vi "Main.vi"() -> ()   [LabVIEW 2020]
doc: "This template is for the Queued Message Handler design pattern.\n\nThe Event Handling Loop generates messages based on user interface actions.\n\nThe Message Handling Loop processes messages generated by the Event Handling Loop, or by other messages. The messages are string values, so new messages can be added easily to the Message Cases case structure in the Message Handling Loop. Each message cluster can also provide an optional value for Message Data, which is a variant that can be converted to whatever message-specific data is required."
uses:
  controls/UI Data.ctl
  controls/Arduino config -- cluster.ctl
  Arduino_stepper/Libraries/Arduino stepper/Support/Motor direction -- enum.ctl
  controls/Camera config parameters -- cluster.ctl
  <vilib>/userdefined/High Color/IMAQdx.ctl
  controls/FGV actions -- enum.ctl
  Arduino_stepper/Libraries/Arduino stepper/Support/COM params--typedef.ctl
  Arduino_stepper/Libraries/Arduino stepper/Support/Motor parameters.ctl
  support/Message Queue/Enqueue Message (Array).vi
  <vilib>/Utility/error.llb/Error Cluster From Error Code.vi
  <vilib>/ErrorRing/Error Ring.xnode
  support/Message Queue/Message Queue.lvlib
  support/User Event - Stop/User Event - Stop.lvlib
  Arduino_stepper/Libraries/Arduino stepper/Arduino stepper.lvlib
  Camera/Libraries/Camera/Camera.lvlib
panel:
  in  "Go to zero":bool
  in  "Mostrar video":bool
  in  "Set zero":bool
  in  "Step 2":dbl=1.0 caption="Paso" format="%#_g°"
  in  "CW Button":bool
  in  "CCW Button":bool
  out "Home?":bool
  in  "To Matlab":bool
  in  "Home":bool
  in  "Step":dbl=5.0 caption="Paso/captura" format="%#_g°"
  out "Image":T1(plugin-control)
  out "Cam connected?":bool
  out "Ard connected?":bool
  out "End-stops":cluster{"ES1":bool, "ES2":bool} caption="Finales de carrera"
  out "Posición actual":dbl format="%#_g°"
  in  "Ángulo":dbl=45.0 caption="Ángulo total" format="%#_g°"
  in  "Stop":bool
  in  "Start acquisition":bool
  in  "Settings":bool
  out "Status":string
  in  "Exit":bool
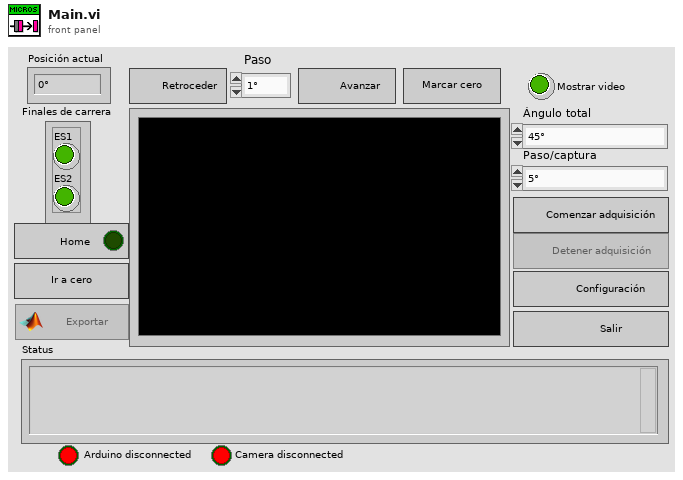
[diagram p1: front panel]
types:
  T1 = typedef "IMAQ Image.ctl" = refnum<image>
  T2 = typedef "UI Data.ctl" = cluster{"Status":string, "Arduino Mod ID":i32, "Arduino config":T3, "Current position":dbl, "End-stops":cluster{"ES1":bool, "ES2":bool}, "Direction":T4, "Camera Mod ID":i32, "Camera config":T5, "System ready?":bool, "Homing?":bool, "Path":path, "Path set?":bool, "Positions":dbl[], "Manual?":bool, "Zero":dbl, "Starting pos":dbl}
  T3 = typedef "Arduino config -- cluster.ctl" = cluster{"VISA resource":refnum<visa-resource-name>}
  T4 = typedef "Arduino stepper.lvlib/Motor direction -- enum.ctl" = enum8{"", "CW", "CCW"}
  T5 = typedef "Camera config parameters -- cluster.ctl" = cluster{"Camera session":T6, "VideoMode":u32}
  T6 = typedef "IMAQdx.ctl" = refnum<k21>
  T7 = typedef "Arduino stepper.lvlib/Broadcast Events--cluster.ctl" = cluster{"Module Did Init":refnum<user-event>, "Status Updated":refnum<user-event>, "Error Reported":refnum<user-event>, "Module Did Stop":refnum<user-event>, "Update Module Execution Status":refnum<user-event>, "Device connected":refnum<user-event>, "Data available":refnum<user-event>, "Info ready":refnum<user-event>, "Connection failed":refnum<user-event>, "Device disconected":refnum<user-event>, "End-position reached":refnum<user-event>, "End-stop reached":refnum<user-event>, "Home reached":refnum<user-event>}
  T8 = typedef "Camera.lvlib/Broadcast Events--cluster.ctl" = cluster{"Module Did Init":refnum<user-event>, "Status Updated":refnum<user-event>, "Error Reported":refnum<user-event>, "Module Did Stop":refnum<user-event>, "Update Module Execution Status":refnum<user-event>, "Helper Loop Status Updated":refnum<user-event>, "Camera connected":refnum<user-event>, "Camera Disconnected":refnum<user-event>, "Image acquired":refnum<user-event>, "Camera acquisition started":refnum<user-event>, "Camera acquisition stopped":refnum<user-event>}
  T9 = typedef "Message Queue.lvlib/All Message Queues.ctl" = cluster{"UI":refnum<queue>}
  T10 = typedef "FGV actions -- enum.ctl" = enum16{"Reset", "Get", "Increment"}
  T11 = enum8{"Enabled", "Disabled", "Disabled and Grayed Out"}
  T12 = typedef "Arduino stepper.lvlib/Motor parameters.ctl" = cluster{"Motor type":enum8{"", "Unipolar", "Bipolar"}, "Direction":T4, "Steps":u16, "Frequency (Hz)":u8, "Step type":enum8{"", "Half", "Full"}}
  T13 = cluster{"Position":i32, "End-stops":cluster{"ES1":bool, "ES2":bool}}
  T14 = typedef "Arduino stepper.lvlib/COM params--typedef.ctl" = cluster{"baud rate":u32, "data bits":u16, "parity":enum16{"None", "Odd", "Even", "Mark", "Space"}, "stop bits":u16, "flow control":u16}
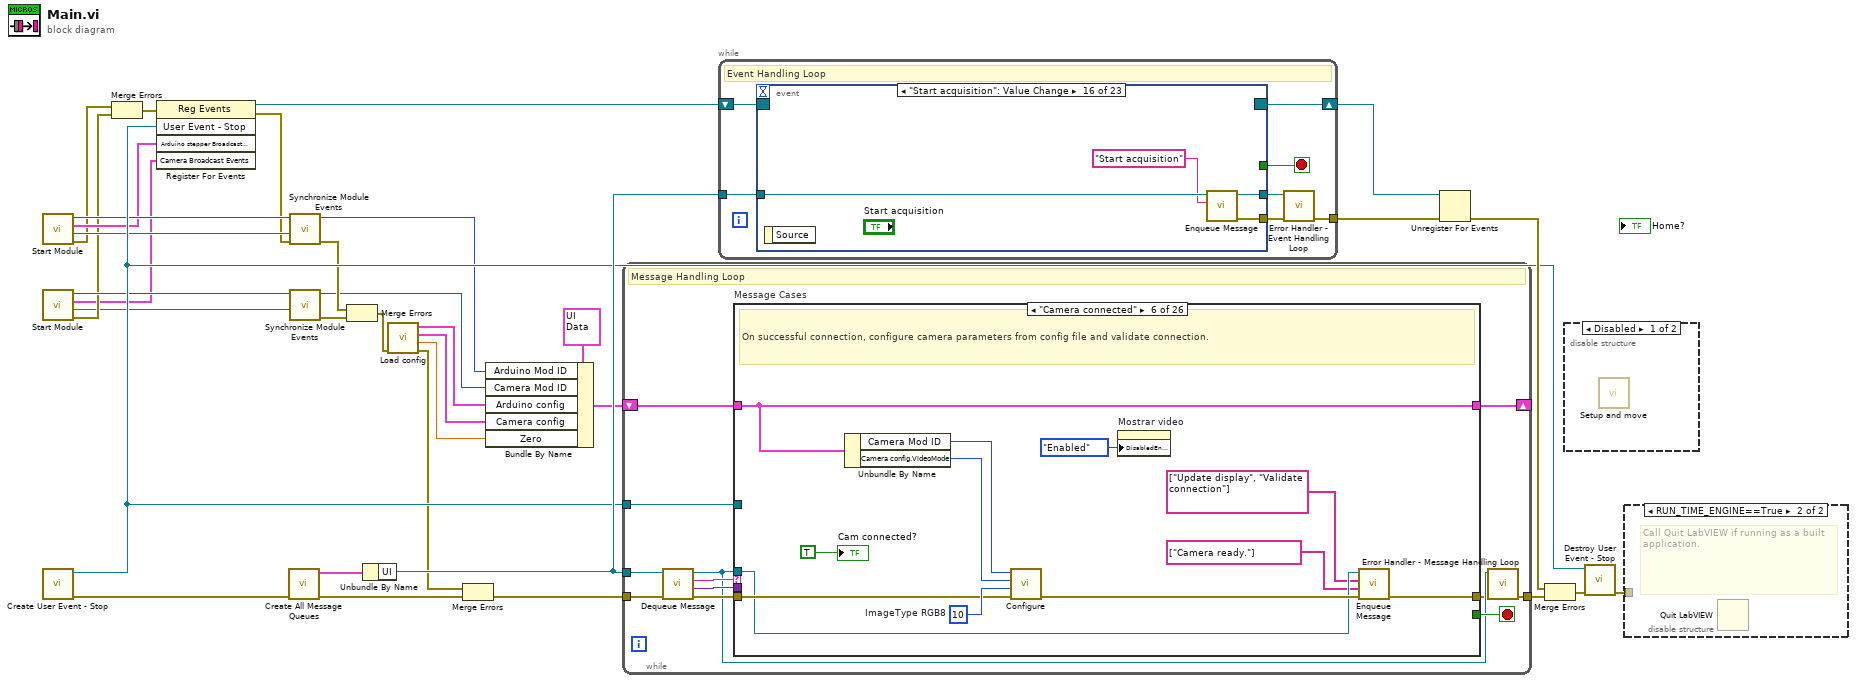
[diagram p0: block diagram]
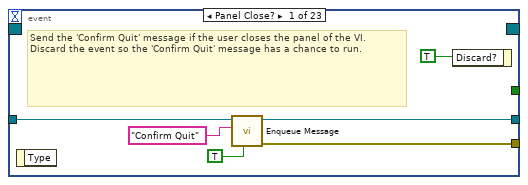
[diagram p4: hidden frame]
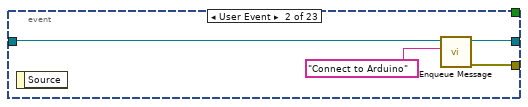
[diagram p5: hidden frame]
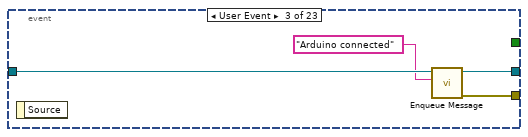
[diagram p6: hidden frame]
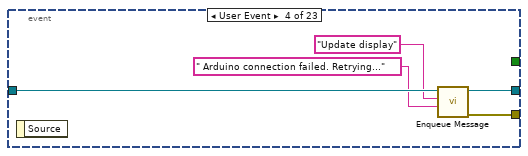
[diagram p7: hidden frame]
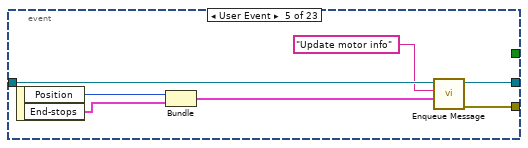
[diagram p8: hidden frame]
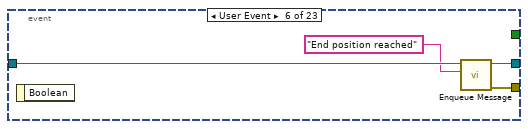
[diagram p9: hidden frame]
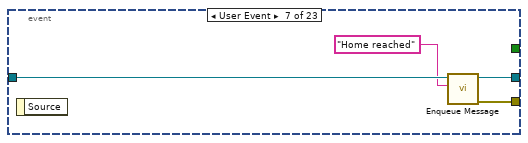
[diagram p10: hidden frame]
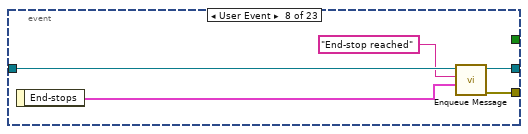
[diagram p11: hidden frame]
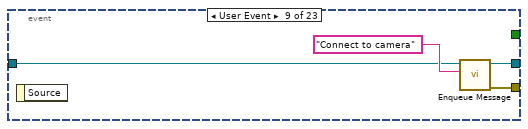
[diagram p12: hidden frame]
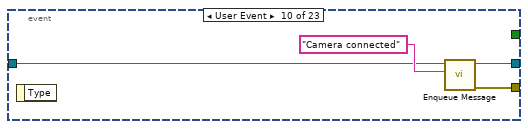
[diagram p13: hidden frame]
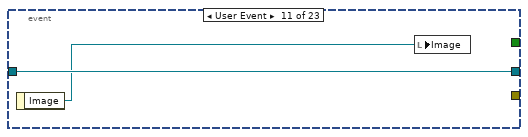
[diagram p14: hidden frame]
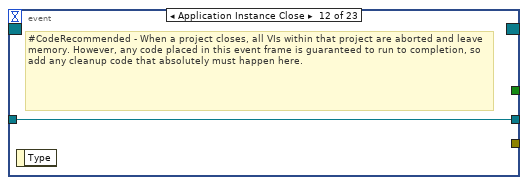
[diagram p15: hidden frame]
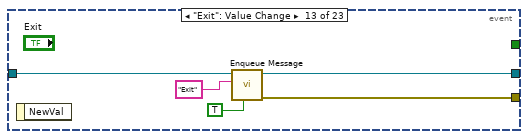
[diagram p16: hidden frame]
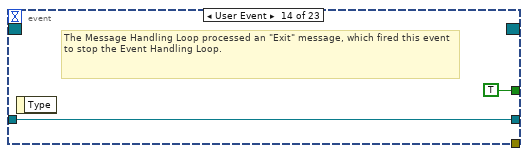
[diagram p17: hidden frame]
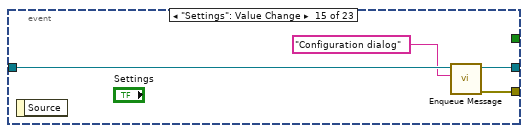
[diagram p18: hidden frame]
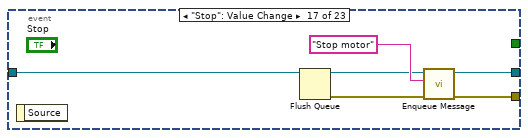
[diagram p19: hidden frame]
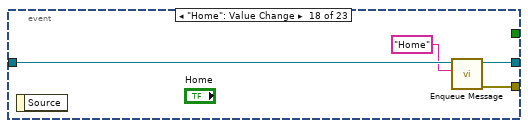
[diagram p20: hidden frame]
diagram:
  n1 = call "Start Module.vi"() -> ("error out"=w9:errorcluster, "Wait for Event Sync?"=w20:bool, "Arduino stepper Broadcast Events"=w21:T7, "Module ID"=w22:i32)  [unwired: 8 in]
  n2 = call "Start Module.vi"() -> ("error out"=w6:errorcluster, "Wait for Event Sync?"=w4:bool, "Camera Broadcast Events"=w5:T8, "Module ID"=w7:i32)  [unwired: 8 in]
  n3 = call "Create User Event - Stop.vi"() -> ("error out"=w31:errorcluster, "User Event - Stop"=w24:refnum<user-event>)  [unwired: 10 in]
  n4 = Merge Errors(w9, w6) -> (w10:errorcluster)
  n5 = register-events(error in=w10, w24, w21, w5) -> (reference out=w25:refnum<event-registration>, error out=w15:errorcluster)  [unwired: 1 in]
  n6 = call "Create All Message Queues.vi"("error in (no error)"=w31) -> ("error out"=w11:errorcluster, "Message Queues out"=w34:T9)  [unwired: 9 in]
  n7 = call "Synchronize Module Events.vi"("error in"=w15, "Wait for Event Sync?"=w20, "Module ID in"=w22) -> ("error out"=w14:errorcluster, "Module ID out"=w17:i32)  [unwired: 7 in]
  n8 = call "Synchronize Module Events.vi"("Wait for Event Sync?"=w4, "Module ID in"=w7) -> ("error out"=w8:errorcluster, "Module ID out"=w3:i32)  [unwired: 8 in]
  n9 = Merge Errors(w14, w8) -> (w13:errorcluster)
  n10 = Unbundle By Name(w34) -> ("UI"=w32:refnum<queue>)
  n11 = call "Load config.vi"("error in (no error)"=w13) -> ("error out"=w12:errorcluster, "Zero"=w1:dbl, "Camera config"=w2:T5, "Arduino config"=w16:T3)  [unwired: 7 in]
  n12 = Merge Errors(w12, w11) -> (w23:errorcluster)
  n13 = Bundle By Name(cluster=T2 {"Status"="", "Arduino Mod ID"=0, "Arduino config"={"VISA resource"=""}, "Current position"=0.0, "End-stops"={"ES1"=FALSE, "ES2"=FALSE}, "Direction"=enum."CW", "Camera Mod ID"=0, "Camera config"={"Camera session"="", "VideoMode"=0}, "System ready?"=FALSE, "Homing?"=FALSE, "Path"=path "", "Path set?"=FALSE, "Positions"=[], "Manual?"=FALSE, "Zero"=0.0, "Starting pos"=0.0} ("Data Cluster"), "Arduino Mod ID"=w17, "Camera Mod ID"=w3, "Arduino config"=w16, "Camera config"=w2, "Zero"=w1) -> (w18:T2)
  n14 = while {
    tunnel: w32 -> [w38]
    shift-right: [w45] -> _
    shift-left: w18 -> [w46]
    tunnel: w24 -> [w43]
    tunnel: w23 -> [w42]
    tunnel: [w36] -> w33
    stop <- w44 stop-if-true
    # "Message Handling Loop"
    n15 = call "Dequeue Message.vi"("error in (no error)"=w42, "Message Queue"=w38) -> ("error out"=w41:errorcluster, "Message Data"=w39:variant, "Message"=w40:string, "dup Message Queue"=w37:refnum<queue>)  [unwired: 6 in]
    n16 = case "Message Cases" shown="\"Camera connected\"" w40 {
      selector: w40 -> [_ _ _ _ _ _ _ _ _ _ _ _ _ _ _ _ _ _ _ _ _ _ _ _ _ w646]
      tunnel: w37 -> [w59 _ w76 w98 w121 w128 w141 w170 w199 w215 _ w283 w321 w371 w387 w415 w464 w497 _ w547 _ _ _ w624 w645 _]
      tunnel: w41 -> [w52 w75 w84 w104 w116 w134 w143 w176 w204 _ w271 w294 w319 w374 w394 w409 w470 w490 w528 w549 w599 w607 w621 w628 w640 _]
      tunnel: [w61 w63 w79 w100 w122 w129 w142 w173 w200 w218 w270 w285 w324 w372 w388 w420 w463 w498 w527 w548 w598 w606 w615 w626 w643 w647] -> w35
      tunnel: w46 -> [w57 w67 w77 w105 w119 w133 w140 w172 w196 w209 w268 w281 w323 w379 w386 w418 w469 w503 w518 w544 w597 w605 w620 w627 w634 w648]
      tunnel: [w56 w65 w77 w105 w118 w133 w137 w171 w195 w217 w269 w280 w322 w379 w385 w417 w468 w502 w517 w543 w597 w605 w620 w627 w634 w648] -> w45
      tunnel: [_ _ _ _ _ _ _ _ _ _ _ _ _ _ _ _ _ _ _ _ _ _ _ _ TRUE _] -> w44
      tunnel: w39 -> [_ w74 _ _ _ _ _ _ _ _ w266 w293 _ _ w392 _ w466 _ _ _ _ w602 w619 _ w637 _]
      tunnel: w43 -> [_ _ _ _ _ _ _ _ _ _ _ _ _ _ _ _ _ _ _ _ _ _ _ _ w642 _]
      frame "Initialize" {
        w49 = FALSE ("System ready?")
        w47 = T11."Disabled and Grayed Out" ("Disabled")
        # "Initialize - All initialization work should take place in this message, since other loops can potentially enqueue messages that execute immediately after this one."
        n17 = call "Image name -- FGV.vi"("error in (no error)"=w52, "Action"=FGV_actions_--_enum."Reset", "Base name"=path "Image_") -> ("error out"=w51:errorcluster)  [unwired: 7 in, 1 out]
        n18 = property on="Start acquisition" class="Bool"("DisabledEnum"=w47) -> ()  [unwired: 2 in, 2 out]
        n19 = property on="To Matlab" class="Bool"("DisabledEnum"=w47) -> ()  [unwired: 2 in, 2 out]
        n20 = property on="Go to zero" class="Bool"("DisabledEnum"=w47) -> ()  [unwired: 2 in, 2 out]
        n21 = property on="Stop" class="Bool"("DisabledEnum"=w47) -> ()  [unwired: 2 in, 2 out]
        n22 = property on="Show/stop video" class="Bool (strict)"("DisabledEnum"=w47, "Value"=FALSE ("Mostrar video")) -> ()  [unwired: 2 in, 2 out]
        n23 = call-poly "Enqueue Message.vi"("error in (no error)"=w51, "Message Data"="Initializing..." ("Initial Message"), "Message"="Update Display", "Message Queue"=w59) -> ("error out"=w61:errorcluster)  [unwired: 6 in, 1 out]
        n24 = Bundle By Name(cluster=w57, "Positions"=dbl[] [0.0], "Current position"=0.0, "Homing?"=w49, "System ready?"=w49, "Path set?"=w49, "Manual?"=w49) -> (w56:T2)
        n25 = local write "Ard connected?"(w49) -> ()
        n26 = local write "Cam connected?"(w49) -> ()
        n27 = local write "Home?"(w49) -> ()
      }
      frame "Update Display" {
        # "Update Display - Convert the message data to a string to display in the Data Display indicator."
        n28 = Variant To Data(error in=w75, type="", Variant=w74) -> (data=w68:string, error out=w64:errorcluster)
        n29 = Unbundle By Name(w67) -> ("Status"=w70:string)
        n30 = Format Date/Time String(time format string (%c)="%d/%m/%y %H:%M:%S%3u") -> (date/time string=w69:string)  [unwired: 2 in]
        n31 = Format Into String(format string="%s: %s\\n", initial string=w70, w69, w68) -> (resulting string=w66:string)  [unwired: 1 in, 1 out]
        "Status" <- w66
        n32 = property on="Status" class="Str"(error in=w64, "Text.Scroll Position"=u32 10000) -> (error out=w63:errorcluster)  [unwired: 1 in, 1 out]
        n33 = Bundle By Name(cluster=w67, "Status"=w66) -> (w65:T2)
      }
      frame "Connect to Arduino" {
        w85 = T14 {"baud rate"=115200, "data bits"=8, "parity"=enum."None", "stop bits"=10, "flow control"=0}  # COM params
        # "Try two reconnections to Arduino. If connection is not successful, call configuration dialog."
        n34 = Unbundle By Name(w77) -> ("Arduino Mod ID"=w78:i32, "Arduino config.VISA resource"=w83:refnum<visa-resource-name>)
        n35 = for {
          N: 2 -> [_]
          tunnel: w85 -> [w96]
          tunnel: w78 -> [w94]
          tunnel: w83 -> [w93]
          shift-right: [w92] -> w80
          shift-left: w84 -> [w95]
          tunnel: [w91] -> w81
          stop <- w91 stop-if-true
          n36 = call "Connect.vi"("error in"=w95, "COM params"=w96, "VISA resource"=w93, "Module ID"=w94) -> ("error out"=w92:errorcluster, "Connected?"=w91:bool)  [unwired: 5 in, 1 out]
        }
        n37 = case shown="False" w81 {
          tunnel: w80 -> [w86 w90]
          tunnel: [w86 w89] -> w79
          tunnel: w78 -> [_ _]
          tunnel: w76 -> [_ w87]
          frame True {
            # "Connection successful."
          }
          frame False {
            # "Could not connect."
            n38 = call-poly "Enqueue Message.vi"("error in (no error)"=w90, "Message"="Configuration dialog", "Message Queue"=w87) -> ("error out"=w89:errorcluster)  [unwired: 7 in, 1 out]
          }
        }
      }
      frame "Connect to camera" {
        w103 = FALSE  # Simulate?
        n39 = Unbundle By Name(w105) -> ("Camera Mod ID"=w101:i32, "Camera config.Camera session"=w97:T6)
        n40 = call "Connect USB.vi"("error in"=w104, "Simulate?"=w103, "Camera session"=w97, "Module ID"=w101) -> ("error out"=w102:errorcluster, "Connected?"=w99:bool)  [unwired: 5 in, 1 out]
        n41 = case shown="False" w99 {
          tunnel: w102 -> [w108 w110]
          tunnel: [w107 w110] -> w100
          tunnel: w98 -> [w106 _]
          frame False {
            # "Connection to camera not made."
            n42 = call-poly "Enqueue Message.vi"("error in (no error)"=w108, "Message"="Configuration dialog", "Message Queue"=w106) -> ("error out"=w107:errorcluster)  [unwired: 7 in, 1 out]
          }
          frame True {
            # "Connection successful."
          }
        }
      }
      frame "Arduino connected" {
        # "On successful connection, update end-stops status and go to validate connection."
        n43 = Unbundle By Name(w119) -> ("Arduino Mod ID"=w120:i32)
        n44 = call "Wait ms.vi"("error in (no error)"=w116, "milliseconds to wait"=u32 100) -> ("error out"=w115:errorcluster)  [unwired: 9 in]
        n45 = call "Read end-stops.vi"("error in"=w115, "Module ID"=w120) -> ("error out"=w123:errorcluster, "End-stops"=w117:cluster{"ES1":bool, "ES2":bool})  [unwired: 7 in, 1 out]
        n46 = local write "End-stops"(w117) -> ()
        n47 = Bundle By Name(cluster=w119, "End-stops"=w117) -> (w118:T2)
        n48 = call-poly "Enqueue Message.vi"("error in (no error)"=w123, "Message Data Array"=string[] ["Arduino ready."] ("Message"), "Message Array"=string[] ["Update display", "Validate connection"] ("Message"), "Message Queue"=w121) -> ("error out"=w122:errorcluster)  [unwired: 6 in, 1 out]
        "Ard connected?" <- TRUE ("Ard connected?")
      }
      frame "Camera connected" {
        w135 = u32 10  # ImageType RGB8
        # "On successful connection, configure camera parameters from config file and validate connection."
        n49 = Unbundle By Name(w133) -> ("Camera Mod ID"=w131:i32, "Camera config.VideoMode"=w132:u32)
        n50 = call "Configure.vi"("error in"=w134, "ImageType"=w135, "VideoMode"=w132, "Module ID"=w131) -> ("error out"=w130:errorcluster)  [unwired: 7 in]
        n51 = property on="Mostrar video" class="Bool (strict)"("DisabledEnum"=T11."Enabled" ("Disabled")) -> ()  [unwired: 2 in, 2 out]
        n52 = call-poly "Enqueue Message.vi"("error in (no error)"=w130, "Message Data Array"=string[] ["Camera ready."] ("Message"), "Message Array"=string[] ["Update display", "Validate connection"] ("Message"), "Message Queue"=w128) -> ("error out"=w129:errorcluster)  [unwired: 6 in, 1 out]
        "Cam connected?" <- TRUE ("Cam connected?")
      }
      frame "Validate connection" {
        # "If both devices connection is successful and system not marked as ready,  set ready flag and home motor position. Otherwise, keep waiting for validation."
        n53 = local read "Cam connected?"() -> (w145:bool)
        n54 = local read "Ard connected?"() -> (w146:bool)
        n55 = Unbundle By Name(w140) -> ("Arduino Mod ID"=w136:i32, "System ready?"=w139:bool)
        n56 = Not(x=w139) -> (.not. x?=w138:bool)
        n57 = Compound Arithmetic op=AND(w138, w146, w145) -> (w144:bool)
        n58 = case shown="True" w144 {
          tunnel: w143 -> [w148 w153]
          tunnel: [w148 w162] -> w142
          tunnel: w141 -> [_ w160]
          tunnel: w140 -> [w147 w157]
          tunnel: [w147 w156] -> w137
          tunnel: w136 -> [_ w149]
          frame False {
          }
          frame True {
            w154 = T11."Disabled and Grayed Out" ("Disabled")
            n59 = call "Read end-stops.vi"("error in"=w153, "Module ID"=w149) -> ("error out"=w152:errorcluster, "End-stops"=w150:cluster{"ES1":bool, "ES2":bool})  [unwired: 7 in, 1 out]
            n60 = property on="Start acquisition" class="Bool"("DisabledEnum"=T11."Enabled" ("Disabled")) -> ()  [unwired: 2 in, 2 out]
            n61 = property on="Home" class="Bool"("DisabledEnum"=w154) -> ()  [unwired: 2 in, 2 out]
            n62 = property on="Stop" class="Bool"(error in=w152, "DisabledEnum"=w154) -> (error out=w151:errorcluster)  [unwired: 1 in, 1 out]
            n63 = Bundle By Name(cluster=w157, "System ready?"=TRUE, "End-stops"=w150) -> (w156:T2)
            n64 = call-poly "Enqueue Message.vi"("error in (no error)"=w151, "Message Data Array"=string[] ["System ready."] ("Message"), "Message Array"=string[] ["Update display", "Home"] ("Message"), "Message Queue"=w160) -> ("error out"=w162:errorcluster)  [unwired: 6 in, 1 out]
          }
        }
      }
      frame "Configuration dialog" {
        n65 = Unbundle By Name(w172) -> ("Camera Mod ID"=w165:i32, "Arduino Mod ID"=w169:i32, "Arduino config"=w175:T3, "Camera config"=w164:T5, "Zero"=w163:dbl)
        n66 = call "Config dialog.vi"("error in (no error)"=w176, "Camera config in"=w164, "Arduino config in"=w175) -> ("error out"=w174:errorcluster, "Cancelled?"=w168:bool, "Camera config out"=w166:T5, "Arduino config out"=w167:T3)  [unwired: 5 in]
        n67 = case shown="False" w168 {
          tunnel: w174 -> [w188 w193]
          tunnel: [w186 w192] -> w173
          tunnel: w170 -> [w185 w191]
          tunnel: w169 -> [w187 _]
          tunnel: w167 -> [w183 _]
          tunnel: w166 -> [w182 _]
          tunnel: w165 -> [w179 _]
          tunnel: w163 -> [w177 _]
          frame False {
            # "Disconnect devices and apply new configuration"
            n68 = call "Disconnect.vi"("error in"=w188, "Module ID"=w187) -> ("error out"=w181:errorcluster)  [unwired: 9 in]
            n69 = call "Disconnect.vi"("error in"=w181, "Module ID"=w179) -> ("error out"=w180:errorcluster)  [unwired: 9 in]
            n70 = call "Save config.vi"("error in (no error)"=w180, "Zero"=w177, "Camera config"=w182, "Arduino config"=w183) -> ("error out"=w184:errorcluster)  [unwired: 7 in]
            n71 = call-poly "Enqueue Message.vi"("error in (no error)"=w184, "Message Array"=string[] ["Connect to Arduino", "Connect to camera"] ("Message"), "Message Queue"=w185) -> ("error out"=w186:errorcluster)  [unwired: 7 in, 1 out]
          }
          frame True {
            # "Config dialog cancelled. Do nothing."
            n72 = call-poly "Enqueue Message.vi"("error in (no error)"=w193, "Message Data"="Configuration cancelled." ("Message"), "Message"="Update display", "Message Queue"=w191) -> ("error out"=w192:errorcluster)  [unwired: 6 in, 1 out]
          }
        }
        n73 = Bundle By Name(cluster=w172, "Arduino config"=w167, "Camera config"=w166) -> (w171:T2)
      }
      frame "Save zero" {
        n74 = Unbundle By Name(w196) -> ("Arduino config"=w203:T3, "Camera config"=w202:T5)
        n75 = local read "Posición actual"() -> (w194:dbl)
        n76 = call "Save config.vi"("error in (no error)"=w204, "Zero"=w194, "Camera config"=w202, "Arduino config"=w203) -> ("error out"=w201:errorcluster)  [unwired: 7 in]
        n77 = Bundle By Name(cluster=w196, "Zero"=w194) -> (w195:T2)
        n78 = call-poly "Enqueue Message.vi"("error in (no error)"=w201, "Message Data"="Starting position updated." ("Message"), "Message"="Update display", "Message Queue"=w199) -> ("error out"=w200:errorcluster)  [unwired: 6 in, 1 out]
      }
      frame "Start acquisition" {
        # "Call file dialog to set a path for all images. If path is not set, do not acquire.\nMove motor only if move conditions are correct. Save first image at 0° of movement."
        n79 = Unbundle By Name(w209) -> ("Arduino Mod ID"=w214:i32, "Camera Mod ID"=w207:i32, "Path"=w212:path, "Path set?"=w210:bool, "End-stops"=w205:cluster{"ES1":bool, "ES2":bool})
        n80 = local read "Home?"() -> (w206:bool)
        n81 = call "Set path.vi"("Path set?"=w210, "Path in"=w212) -> ("error out"=w213:errorcluster, "cancelled?"=w211:bool, "Path out"=w208:path)  [unwired: 7 in]
        n82 = case shown="False" w211 {
          tunnel: [w235 w256] -> w218
          tunnel: [w234 w252] -> w217
          tunnel: Motor_direction_--_enum."CCW" ("Direction") -> [w232 _]
          tunnel: w215 -> [w231 w255]
          tunnel: w214 -> [w228 _]
          tunnel: w213 -> [w227 w257]
          tunnel: w209 -> [w226 w252]
          tunnel: w208 -> [w223 _]
          tunnel: w207 -> [w222 _]
          tunnel: w206 -> [w221 _]
          tunnel: w205 -> [w219 _]
          frame False {
            # "Path is set correctly. Start aquisition."
            n83 = Bundle By Name(cluster=w226, "Path"=w223, "Path set?"=TRUE, "Manual?"=FALSE) -> (w224:T2)
            n84 = call "Check move conditions.vi"("Is Home?"=w221, "error in (no error)"=w227, "End-stops"=w219, "Direction"=w232) -> ("error out"=w233:errorcluster, "String"=w229:string, "Move?"=w230:bool)  [unwired: 5 in]
            n85 = case shown="True" w230 {
              tunnel: [w241 w251] -> w235
              tunnel: w228 -> [_ _]
              tunnel: [w236 w245] -> w234
              tunnel: w233 -> [w240 w250]
              tunnel: w232 -> [_ w247]
              tunnel: w231 -> [w239 w249]
              tunnel: w229 -> [w237 _]
              tunnel: w224 -> [w236 w246]
              tunnel: w222 -> [_ _]
              frame False {
                # "Move conditions not met"
                n86 = call-poly "Enqueue Message.vi"("error in (no error)"=w240, "Message Data"=w237, "Message"="Update Display", "Message Queue"=w239) -> ("error out"=w241:errorcluster)  [unwired: 6 in, 1 out]
              }
              frame True {
                # "Start moving"
                n87 = local read "Posición actual"() -> (w242:dbl)
                n88 = Build Array(w242) -> (w243:dbl[])
                n89 = Bundle By Name(cluster=w246, "End-stops"=cluster{"ES1":bool, "ES2":bool} {"ES1"=FALSE, "ES2"=FALSE}, "Positions"=w243, "Starting pos"=w242) -> (w245:T2)
                n90 = call-poly "Enqueue Message.vi"("error in (no error)"=w250, "Message Data"=w247, "Message"="Begin movement", "Message Queue"=w249) -> ("error out"=w251:errorcluster)  [unwired: 6 in, 1 out]
              }
            }
          }
          frame True {
            # "Path not set. Do nothing."
            n91 = call-poly "Enqueue Message.vi"("error in (no error)"=w257, "Message Data"="Path not selected or empty. Stopping acquisition." ("Message"), "Message"="Update Display", "Message Queue"=w255) -> ("error out"=w256:errorcluster)  [unwired: 6 in, 1 out]
          }
        }
      }
      frame "Begin movement" {
        w274 = T11."Enabled" ("Disabled")
        w259 = T11."Disabled and Grayed Out" ("Disabled")
        n92 = Variant To Data(error in=w271, type=Motor_direction_--_enum."CCW" ("Direction"), Variant=w266) -> (data=w264:T4, error out=w261:errorcluster)
        n93 = Unbundle By Name(w268) -> ("Arduino Mod ID"=w267:i32, "Path"=w262:path, "Camera Mod ID"=w260:i32)
        n94 = call "Get and save image.vi"("error in (no error)"=w261, "Camera Mod ID"=w260, "Path"=w262) -> ("error out"=w276:errorcluster, "Image out"=→"Image":T1)  [unwired: 7 in]
        n95 = call "Setup and move.vi"("Motor params"=T12 {"Motor type"=enum."Unipolar", "Direction"=enum."CW", "Steps"=1000, "Frequency (Hz)"=127, "Step type"=enum."Full"}, "error in (no error)"=w276, "Ángulo"="Step", "Direction"=w264, "Arduino Mod ID"=w267) -> ("error out"=w270:errorcluster)  [unwired: 6 in]
        n96 = Bundle By Name(cluster=w268, "Homing?"=FALSE, "Direction"=w264) -> (w269:T2)
        n97 = local write "Home?"(FALSE ("Home?")) -> ()
        n98 = property on="Home" class="Bool"("DisabledEnum"=w274) -> ()  [unwired: 2 in, 2 out]
        n99 = property on="Stop" class="Bool"("DisabledEnum"=w274) -> ()  [unwired: 2 in, 2 out]
        n100 = property on="Start acquisition" class="Bool"("DisabledEnum"=w259) -> ()  [unwired: 2 in, 2 out]
        n101 = property on="Mostrar video" class="Bool (strict)"("DisabledEnum"=w259, "Value"=FALSE ("Mostrar video")) -> ()  [unwired: 2 in, 2 out]
      }
      frame "Jog" {
        n102 = Unbundle By Name(w281) -> ("Arduino Mod ID"=w287:i32, "End-stops"=w278:cluster{"ES1":bool, "ES2":bool})
        n103 = Variant To Data(error in=w294, type=Motor_direction_--_enum."CW" ("Direction"), Variant=w293) -> (data=w286:T4, error out=w292:errorcluster)
        n104 = disable-structure shown="Enabled" {
          disable-tunnel: w292 -> [w298 _]
          disable-tunnel: [w297 _] -> w291
          disable-tunnel: w287 -> [w296 _]
          disable-tunnel: [w295 w299] -> w279
          disable-tunnel: w278 -> [_ w299]
          frame Disabled {
            n105 = call "Read end-stops.vi"("error in"=w298, "Module ID"=w296) -> ("error out"=w297:errorcluster, "End-stops"=w295:cluster{"ES1":bool, "ES2":bool})  [unwired: 7 in, 1 out]
          }
          frame Enabled {
          }
        }
        n106 = local read "Home?"() -> (w282:bool)
        n107 = call "Check move conditions.vi"("Is Home?"=w282, "error in (no error)"=w291, "End-stops"=w279, "Direction"=w286) -> ("error out"=w288:errorcluster, "String"=w284:string, "Move?"=w289:bool)  [unwired: 5 in]
        n108 = case shown="True" w289 {
          tunnel: w288 -> [w304 w316]
          tunnel: w287 -> [_ w315]
          tunnel: w286 -> [_ w311]
          tunnel: [w305 w313] -> w285
          tunnel: w284 -> [w303 _]
          tunnel: w283 -> [w301 _]
          tunnel: w281 -> [w300 w308]
          tunnel: [w300 w312] -> w280
          frame False {
            n109 = call-poly "Enqueue Message.vi"("error in (no error)"=w304, "Message Data"=w303, "Message"="Update Display", "Message Queue"=w301) -> ("error out"=w305:errorcluster)  [unwired: 6 in, 1 out]
          }
          frame True {
            w306 = T11."Enabled" ("Disabled")
            n110 = call "Setup and move.vi"("Motor params"=T12 {"Motor type"=enum."Unipolar", "Direction"=enum."CW", "Steps"=1000, "Frequency (Hz)"=127, "Step type"=enum."Full"}, "error in (no error)"=w316, "Ángulo"="Step 2", "Direction"=w311, "Arduino Mod ID"=w315) -> ("error out"=w313:errorcluster)  [unwired: 6 in]
            n111 = property on="Home" class="Bool"("DisabledEnum"=w306) -> ()  [unwired: 2 in, 2 out]
            n112 = property on="Go to zero" class="Bool"("DisabledEnum"=w306) -> ()  [unwired: 2 in, 2 out]
            n113 = Bundle By Name(cluster=w308, "Manual?"=TRUE, "Direction"=w311, "End-stops"=cluster{"ES1":bool, "ES2":bool} {"ES1"=FALSE, "ES2"=FALSE}) -> (w312:T2)
            n114 = local write "Home?"(FALSE ("Home?")) -> ()
          }
        }
      }
      frame "Home" {
        # "If move conditions are met, move in CW direction 90 degrees or until ES1 is reached."
        n115 = Unbundle By Name(w323) -> ("Arduino Mod ID"=w320:i32)
        n116 = local read "Home?"() -> (w318:bool)
        n117 = disable-structure shown="Enabled" {
          disable-tunnel: [w337 w358] -> w324
          disable-tunnel: w323 -> [w336 w362]
          disable-tunnel: [w335 w360] -> w322
          disable-tunnel: w321 -> [w333 w357]
          disable-tunnel: w320 -> [w328 w363]
          disable-tunnel: w319 -> [w326 w368]
          disable-tunnel: w318 -> [w325 _]
          frame Disabled {
            w327 = Motor_direction_--_enum."CW" ("Direction")
            n118 = call "Read end-stops.vi"("error in"=w326, "Module ID"=w328) -> ("error out"=w330:errorcluster, "End-stops"=w329:cluster{"ES1":bool, "ES2":bool})  [unwired: 7 in, 1 out]
            n119 = call "Check move conditions.vi"("Is Home?"=w325, "error in (no error)"=w330, "End-stops"=w329, "Direction"=w327) -> ("error out"=w334:errorcluster, "String"=w331:string, "Move?"=w332:bool)  [unwired: 5 in]
            n120 = case shown="True" w332 {
              tunnel: [w342 w354] -> w337
              tunnel: w328 -> [_ w353]
              tunnel: w336 -> [w343 w352]
              tunnel: [w343 w351] -> w335
              tunnel: w334 -> [w341 w350]
              tunnel: w327 -> [_ w349]
              tunnel: w333 -> [w340 _]
              tunnel: w331 -> [w338 _]
              frame False {
                # "Move conditions not met"
                n121 = call-poly "Enqueue Message.vi"("error in (no error)"=w341, "Message Data"=w338, "Message"="Update Display", "Message Queue"=w340) -> ("error out"=w342:errorcluster)  [unwired: 6 in, 1 out]
              }
              frame True {
                w344 = 90.0  # Max angle
                # "Start moving"
                n122 = call "Setup and move.vi"("Motor params"=T12 {"Motor type"=enum."Unipolar", "Direction"=enum."CW", "Steps"=1000, "Frequency (Hz)"=255, "Step type"=enum."Full"}, "error in (no error)"=w350, "Ángulo"=w344, "Direction"=w349, "Arduino Mod ID"=w353) -> ("error out"=w354:errorcluster)  [unwired: 6 in]
                n123 = Bundle By Name(cluster=w352, "Direction"=w349, "Homing?"=TRUE) -> (w351:T2)
                n124 = property on="Start acquisition" class="Bool"("DisabledEnum"=T11."Disabled and Grayed Out" ("Disabled")) -> ()  [unwired: 2 in, 2 out]
                n125 = property on="Stop" class="Bool"("DisabledEnum"=T11."Enabled" ("Disabled")) -> ()  [unwired: 2 in, 2 out]
              }
            }
          }
          frame Enabled {
            w365 = 50  # Timeout
            n126 = call "Home.vi"("error in"=w368, "Module ID"=w363) -> ("error out"=w364:errorcluster)  [unwired: 9 in]
            n127 = Bundle By Name(cluster=w362, "Homing?"=TRUE) -> (w360:T2)
            n128 = call "Read port continuously.vi"("error in"=w364, "Timeout"=w365, "Module ID"=w363) -> ("error out"=w359:errorcluster)  [unwired: 8 in]
            n129 = call-poly "Enqueue Message.vi"("error in (no error)"=w359, "Message Data"="Homing..." ("Message"), "Message"="Update Display", "Message Queue"=w357) -> ("error out"=w358:errorcluster)  [unwired: 6 in, 1 out]
            n130 = property on="Start acquisition" class="Bool"("DisabledEnum"=T11."Disabled and Grayed Out" ("Disabled")) -> ()  [unwired: 2 in, 2 out]
            n131 = property on="Stop" class="Bool"("DisabledEnum"=T11."Enabled" ("Disabled")) -> ()  [unwired: 2 in, 2 out]
          }
        }
      }
      frame "Stop motor" {
        n132 = Unbundle By Name(w379) -> ("Arduino Mod ID"=w375:i32)
        n133 = call "Stop continuous reading.vi"("error in"=w374, "Module ID"=w375) -> ("error out"=w376:errorcluster)  [unwired: 9 in]
        n134 = call "Stop motor.vi"("error in"=w376, "Module ID"=w375) -> ("error out"=w373:errorcluster)  [unwired: 9 in]
        n135 = property on="Stop" class="Bool"("DisabledEnum"=T11."Disabled and Grayed Out" ("Disabled")) -> ()  [unwired: 2 in, 2 out]
        n136 = property on="Start acquisition" class="Bool"("DisabledEnum"=T11."Enabled" ("Disabled")) -> ()  [unwired: 2 in, 2 out]
        n137 = call-poly "Enqueue Message.vi"("error in (no error)"=w373, "Message Data"="Stop sent by user." ("Message"), "Message"="Update Display", "Message Queue"=w371) -> ("error out"=w372:errorcluster)  [unwired: 6 in, 1 out]
      }
      frame "Update motor info" {
        # "Get End-stop and position info from continous reading. If and end-stop is reached, stop movement."
        n138 = Variant To Data(error in=w394, type=T13 {"Position"=0, "End-stops"={"ES1"=FALSE, "ES2"=FALSE}} ("output cluster"), Variant=w392) -> (data=w391:T13, error out=w383:errorcluster)
        n139 = Unbundle By Name(w386) -> ("Current position"=w389:dbl, "Direction"=w380:T4)
        n140 = Unbundle By Name(w391) -> ("Position"=w390:i32, "End-stops"=w381:cluster{"ES1":bool, "ES2":bool})
        "End-stops" <- w381
        n141 = call "Calculate new position.vi"("error in (no error)"=w383, "Position from motor"=w390, "Direction"=w380, "Current position in"=w389) -> ("error out"=w382:errorcluster, "Position out"=w384:dbl)  [unwired: 6 in]
        "Posición actual" <- w384
        n142 = disable-structure shown="Enabled" {
          disable-tunnel: [w402 w408] -> w388
          disable-tunnel: w387 -> [w401 _]
          disable-tunnel: w382 -> [w400 w408]
          disable-tunnel: w381 -> [w399 _]
          disable-tunnel: w380 -> [w398 _]
          frame Disabled {
            n143 = local read "Home?"() -> (w395:bool)
            n144 = call "Check move conditions.vi"("Is Home?"=w395, "error in (no error)"=w400, "End-stops"=w399, "Direction"=w398) -> ("error out"=w397:errorcluster, "Move?"=w396:bool)  [unwired: 5 in, 1 out]
            n145 = case shown="True" w396 {
              tunnel: w397 -> [w403 w407]
              tunnel: [w405 w407] -> w402
              tunnel: w401 -> [w404 _]
              frame False {
                # "End-stop reached."
                n146 = call-poly "Enqueue Message.vi"("error in (no error)"=w403, "Message"="Stop motor", "Message Queue"=w404) -> ("error out"=w405:errorcluster)  [unwired: 7 in, 1 out]
              }
              frame True {
                # "Keep moving"
              }
            }
          }
          frame Enabled {
          }
        }
        n147 = Bundle By Name(cluster=w386, "Current position"=w384, "End-stops"=w381) -> (w385:T2)
      }
      frame "End position reached" {
        # "If end-position is reached, stop motor. If the motor is homing, change disable state of controls, otherwise check move condition."
        n148 = Unbundle By Name(w418) -> ("Manual?"=w414:bool, "Camera Mod ID"=w413:i32, "Arduino Mod ID"=w412:i32, "Homing?"=w419:bool, "Path"=w416:path)
        n149 = call "Stop continuous reading.vi"("error in"=w409, "Module ID"=w412) -> ("error out"=w410:errorcluster)  [unwired: 9 in]
        n150 = call "Stop motor.vi"("error in"=w410, "Module ID"=w412) -> ("error out"=w411:errorcluster)  [unwired: 9 in]
        n151 = case shown="False" w414 {
          tunnel: [w427 w450] -> w420
          tunnel: w419 -> [w426 _]
          tunnel: w418 -> [w425 w455]
          tunnel: [w424 w454] -> w417
          tunnel: w416 -> [_ _]
          tunnel: w415 -> [w423 _]
          tunnel: w411 -> [w422 w450]
          tunnel: w412 -> [w421 _]
          tunnel: w413 -> [_ _]
          frame False {
            # "Automatic movement. Check move conditions."
            n152 = case shown="False" w426 {
              tunnel: w422 -> [w429 w441]
              tunnel: [w436 w449] -> w427
              tunnel: w425 -> [w432 w446]
              tunnel: [w431 w444] -> w424
              tunnel: w423 -> [w435 w442]
              tunnel: w421 -> [_ _]
              frame False {
                # "Partial end-position. Check if system needs to keep moving."
                n153 = Unbundle By Name(w432) -> ("Positions"=w434:dbl[], "Current position"=w433:dbl)
                n154 = local read "Posición actual"() -> (w428:dbl)
                n155 = Build Array (concatenate)(w434, w433) -> (w430:dbl[])
                n156 = Bundle By Name(cluster=w432, "Positions"=w430, "Current position"=w428) -> (w431:T2)
                n157 = call-poly "Enqueue Message.vi"("error in (no error)"=w429, "Message Data Array"=string[] ["End-position reached."] ("Message"), "Message Array"=string[] ["Update Display", "Check move condition"] ("Message"), "Message Queue"=w435) -> ("error out"=w436:errorcluster)  [unwired: 6 in, 1 out]
              }
              frame True {
                w440 = T11."Enabled" ("Disabled")
                w443 = T11."Disabled and Grayed Out" ("Disabled")
                # "Zero position reached."
                n158 = property on="Start acquisition" class="Bool"("DisabledEnum"=w440) -> ()  [unwired: 2 in, 2 out]
                n159 = property on="Mostrar video" class="Bool (strict)"("DisabledEnum"=w440) -> ()  [unwired: 2 in, 2 out]
                n160 = property on="Home" class="Bool"("DisabledEnum"=w443) -> ()  [unwired: 2 in, 2 out]
                n161 = property on="Stop" class="Bool"("DisabledEnum"=w443) -> ()  [unwired: 2 in, 2 out]
                n162 = local read "Posición actual"() -> (w439:dbl)
                n163 = Bundle By Name(cluster=w446, "Homing?"=FALSE, "Current position"=w439) -> (w444:T2)
                n164 = call-poly "Enqueue Message.vi"("error in (no error)"=w441, "Message Data"="Zero position reached." ("Message"), "Message"="Update Display", "Message Queue"=w442) -> ("error out"=w449:errorcluster)  [unwired: 6 in, 1 out]
              }
            }
          }
          frame True {
            w451 = T11."Enabled" ("Disabled")
            # "Manual movement. Do nothing."
            n165 = Unbundle By Name(w455) -> ("Current position"=w453:dbl)
            n166 = Build Array(w453) -> (w452:dbl[])
            n167 = property on="Mostrar video" class="Bool (strict)"("DisabledEnum"=w451) -> ()  [unwired: 2 in, 2 out]
            n168 = property on="Start acquisition" class="Bool"("DisabledEnum"=w451) -> ()  [unwired: 2 in, 2 out]
            n169 = Bundle By Name(cluster=w455, "Positions"=w452) -> (w454:T2)
          }
        }
      }
      frame "End-stop reached" {
        n170 = Unbundle By Name(w469) -> ("Arduino Mod ID"=w467:i32, "Direction"=w461:T4)
        n171 = Variant To Data(error in=w470, type=cluster{"ES1":bool, "ES2":bool} {"ES1"=FALSE, "ES2"=FALSE} ("End-stops"), Variant=w466) -> (data=w456:cluster{"ES1":bool, "ES2":bool}, error out=w462:errorcluster)
        n172 = local write "End-stops"(w456) -> ()
        n173 = local read "Home?"() -> (w460:bool)
        n174 = call "Check move conditions.vi"("Is Home?"=w460, "error in (no error)"=w462, "End-stops"=w456, "Direction"=w461) -> ("error out"=w459:errorcluster, "String"=w457:string, "Move?"=w458:bool)  [unwired: 5 in]
        n175 = case shown="False" w458 {
          tunnel: w469 -> [w482 w486]
          tunnel: [w481 w486] -> w468
          tunnel: w467 -> [w480 _]
          tunnel: w464 -> [w479 _]
          tunnel: [w478 w485] -> w463
          tunnel: w459 -> [w473 w485]
          tunnel: w457 -> [w475 _]
          tunnel: w456 -> [w474 _]
          frame False {
            w483 = T11."Enabled" ("Disabled")
            # "End-stop (not home) reached. Stop motor."
            n176 = call "Stop continuous reading.vi"("error in"=w473, "Module ID"=w480) -> ("error out"=w472:errorcluster)  [unwired: 9 in]
            n177 = call "Stop motor.vi"("error in"=w472, "Module ID"=w480) -> ("error out"=w471:errorcluster)  [unwired: 9 in]
            n178 = Bundle By Name(cluster=w482, "Path set?"=FALSE, "End-stops"=w474) -> (w481:T2)
            n179 = call-poly "Enqueue Message.vi"("error in (no error)"=w471, "Message Data"=w475, "Message"="Update Display", "Message Queue"=w479) -> ("error out"=w478:errorcluster)  [unwired: 6 in, 1 out]
            n180 = property on="Stop" class="Bool"("DisabledEnum"=T11."Disabled and Grayed Out" ("Disabled")) -> ()  [unwired: 2 in, 2 out]
            n181 = property on="Home" class="Bool"("DisabledEnum"=w483) -> ()  [unwired: 2 in, 2 out]
            n182 = property on="Mostrar video" class="Bool (strict)"("DisabledEnum"=w483) -> ()  [unwired: 2 in, 2 out]
            n183 = property on="Start acquisition" class="Bool"("DisabledEnum"=w483) -> ()  [unwired: 2 in, 2 out]
          }
          frame True {
            # "End-stop reported is Home end-stop. Keep moving if movement is CCW."
          }
        }
      }
      frame "Home reached" {
        w504 = 0.0 ("Current position")
        w499 = T11."Enabled" ("Disabled")
        w500 = T11."Disabled and Grayed Out" ("Disabled")
        n184 = Unbundle By Name(w503) -> ("Arduino Mod ID"=w491:i32)  [unwired: 1 out]
        n185 = call "Stop motor.vi"("error in"=w490, "Module ID"=w491) -> ("error out"=w489:errorcluster)  [unwired: 9 in]
        n186 = call "Stop continuous reading.vi"("error in"=w489, "Module ID"=w491) -> ("error out"=w488:errorcluster)  [unwired: 9 in]
        n187 = call "Image name -- FGV.vi"("error in (no error)"=w488, "Action"=FGV_actions_--_enum."Reset") -> ("error out"=w493:errorcluster)  [unwired: 8 in, 1 out]
        n188 = local write "Home?"(TRUE ("Home?")) -> ()
        n189 = disable-structure shown="Disabled" {
          disable-tunnel: w493 -> [w512 w513]
          disable-tunnel: [w511 w513] -> w492
          disable-tunnel: w491 -> [w510 _]
          frame Disabled {
            n190 = call "Setup and move.vi"("Motor params"=T12 {"Motor type"=enum."Unipolar", "Direction"=enum."CW", "Steps"=100, "Frequency (Hz)"=127, "Step type"=enum."Full"}, "error in (no error)"=w512, "Ángulo"=1.0, "Direction"=Motor_direction_--_enum."CW", "Arduino Mod ID"=w510) -> ("error out"=w511:errorcluster)  [unwired: 6 in]
          }
          frame Enabled {
          }
        }
        n191 = Bundle By Name(cluster=w503, "Positions"=dbl[] [0.0], "Manual?"=FALSE, "Current position"=w504) -> (w502:T2)
        n192 = local write "Posición actual"(w504) -> ()
        n193 = property on="Go to zero" class="Bool"("DisabledEnum"=T11."Enabled" ("Disabled")) -> ()  [unwired: 2 in, 2 out]
        n194 = call-poly "Enqueue Message.vi"("error in (no error)"=w492, "Message Data"="Home position reached." ("Message"), "Message"="Update Display", "Message Queue"=w497) -> ("error out"=w498:errorcluster)  [unwired: 6 in, 1 out]
        n195 = property on="Mostrar video" class="Bool (strict)"("DisabledEnum"=w499) -> ()  [unwired: 2 in, 2 out]
        n196 = property on="Start acquisition" class="Bool"("DisabledEnum"=w499) -> ()  [unwired: 2 in, 2 out]
        n197 = property on="Stop" class="Bool"("DisabledEnum"=w500) -> ()  [unwired: 2 in, 2 out]
        n198 = property on="Home" class="Bool"("DisabledEnum"=w500) -> ()  [unwired: 2 in, 2 out]
      }
      frame "Go to zero" {
        w514 = T11."Disabled and Grayed Out" ("Disabled")
        # "#TODO: Disable controls."
        n199 = Unbundle By Name(w518) -> ("Arduino Mod ID"=w520:i32, "Current position"=w529:dbl, "Zero"=w522:dbl)
        n200 = Subtract(x=w529, y=w522) -> (x-y=w519:dbl)
        n201 = Absolute Value(x=w519) -> (abs(x)=w521:dbl)
        n202 = Greater Than 0?(x=w519) -> (x > 0?=w525:bool)
        n203 = Select(t=Motor_direction_--_enum."CW" ("Direction"), s=w525, f=Motor_direction_--_enum."CCW" ("Direction")) -> (s? t:f=w516:T4)
        n204 = call "Setup and move.vi"("Motor params"=T12 {"Motor type"=enum."Unipolar", "Direction"=enum."CW", "Steps"=100, "Frequency (Hz)"=127, "Step type"=enum."Full"}, "error in (no error)"=w528, "Ángulo"=w521, "Direction"=w516, "Arduino Mod ID"=w520) -> ("error out"=w527:errorcluster)  [unwired: 6 in]
        n205 = Bundle By Name(cluster=w518, "Direction"=w516) -> (w517:T2)
        n206 = property on="Start acquisition" class="Bool"("DisabledEnum"=w514) -> ()  [unwired: 2 in, 2 out]
        n207 = property on="Go to zero" class="Bool"("DisabledEnum"=w514) -> ()  [unwired: 2 in, 2 out]
        n208 = property on="Stop" class="Bool"("DisabledEnum"=T11."Enabled" ("Disabled")) -> ()  [unwired: 2 in, 2 out]
      }
      frame "Check move condition" {
        n209 = Unbundle By Name(w544) -> ("Path"=w545:path, "Positions"=w546:dbl[], "Camera Mod ID"=w535:i32, "Arduino Mod ID"=w538:i32, "Direction"=w537:T4, "End-stops"=w536:cluster{"ES1":bool, "ES2":bool}, "Current position"=w533:dbl, "Starting pos"=w530:dbl)
        n210 = local read "Home?"() -> (w542:bool)
        n211 = Add(x=w530, y="Ángulo") -> (x+y=w531:dbl)
        n212 = Subtract(x=w533, y=w531) -> (x-y=w540:dbl)
        n213 = In Range and Coerce(upper limit=0.2, x=w540, lower limit=-0.2) -> (In Range?=w541:bool)  [unwired: 1 out]
        n214 = case shown="False" w541 {
          tunnel: w549 -> [w558 w590]
          tunnel: [w560 w594] -> w548
          tunnel: w538 -> [w551 w589]
          tunnel: w547 -> [w559 w588]
          tunnel: w537 -> [w550 _]
          tunnel: w546 -> [_ w587]
          tunnel: w545 -> [_ w577]
          tunnel: w544 -> [w555 w584]
          tunnel: [w555 w582] -> w543
          tunnel: w542 -> [w554 _]
          tunnel: w536 -> [w552 _]
          tunnel: w535 -> [_ w576]
          frame False {
            # "Move again."
            n215 = call "Check move conditions.vi"("Is Home?"=w554, "error in (no error)"=w558, "End-stops"=w552, "Direction"=w550) -> ("error out"=w557:errorcluster, "String"=w553:string, "Move?"=w556:bool)  [unwired: 5 in]
            n216 = case shown="False" w556 {
              tunnel: [w569 w574] -> w560
              tunnel: w559 -> [w568 w572]
              tunnel: w557 -> [w566 w571]
              tunnel: w553 -> [w562 _]
              tunnel: w551 -> [w561 _]
              tunnel: w550 -> [_ w570]
              frame False {
                n217 = call "Stop continuous reading.vi"("error in"=w566, "Module ID"=w561) -> ("error out"=w564:errorcluster)  [unwired: 9 in]
                n218 = call "Image name -- FGV.vi"("error in (no error)"=w564, "Action"=FGV_actions_--_enum."Reset") -> ("error out"=w563:errorcluster)  [unwired: 8 in, 1 out]
                n219 = call-poly "Enqueue Message.vi"("error in (no error)"=w563, "Message Data"=w562, "Message"="Update display", "Message Queue"=w568) -> ("error out"=w569:errorcluster)  [unwired: 6 in, 1 out]
              }
              frame True {
                n220 = call-poly "Enqueue Message.vi"("error in (no error)"=w571, "Message Data"=w570, "Message"="Begin movement", "Message Queue"=w572) -> ("error out"=w574:errorcluster)  [unwired: 6 in, 1 out]
              }
            }
          }
          frame True {
            w585 = T11."Enabled" ("Disabled")
            # "End of movement"
            n221 = call "Stop continuous reading.vi"("error in"=w590, "Module ID"=w589) -> ("error out"=w579:errorcluster)  [unwired: 9 in]
            n222 = call "Get and save image.vi"("error in (no error)"=w579, "Camera Mod ID"=w576, "Path"=w577) -> ("error out"=w578:errorcluster, "Image out"=w575:T1)  [unwired: 7 in]
            n223 = call "Image name -- FGV.vi"("error in (no error)"=w578, "Action"=FGV_actions_--_enum."Reset") -> ("error out"=w581:errorcluster)  [unwired: 8 in, 1 out]
            n224 = local write "Image"(w575) -> ()
            n225 = property on="Stop" class="Bool"("DisabledEnum"=T11."Disabled and Grayed Out" ("Disabled")) -> ()  [unwired: 2 in, 2 out]
            n226 = property on="Start acquisition" class="Bool"("DisabledEnum"=w585) -> ()  [unwired: 2 in, 2 out]
            n227 = property on="To Matlab" class="Bool"("DisabledEnum"=w585) -> ()  [unwired: 2 in, 2 out]
            n228 = call "Save reference file -- subVI.vi"("error in (no error)"=w581, "Positions"=w587, "Path"=w577) -> ("error out"=w586:errorcluster)  [unwired: 8 in]
            n229 = Bundle By Name(cluster=w584, "Path set?"=FALSE) -> (w582:T2)
            n230 = call-poly "Enqueue Message.vi"("error in (no error)"=w586, "Message Data Array"=string[] ["Acquisition complete. Homing..."] ("Message Array"), "Message Array"=string[] ["Update Display", "Home"], "Message Queue"=w588) -> ("error out"=w594:errorcluster)  [unwired: 6 in, 1 out]
          }
        }
      }
      frame "Export to Matlab" {
        w595 = TRUE  # Display?
        n231 = Unbundle By Name(w597) -> ("Path"=w596:path)
        n232 = call "Export to Matlab.vi"("Display?"=w595, "error in (no error)"=w599, "Log file path"=w596) -> ("error out"=w598:errorcluster)  [unwired: 8 in]
      }
      frame "Toggle video on/off" {
        n233 = Variant To Data(error in=w607, type="", Variant=w602) -> (data=w600:string, error out=w603:errorcluster)
        n234 = Unbundle By Name(w605) -> ("Camera Mod ID"=w604:i32)
        n235 = case shown="\"Stop video\", Default" w600 {
          tunnel: [w609 w614] -> w606
          tunnel: w604 -> [w608 w613]
          tunnel: w603 -> [w610 w611]
          frame "Stop video", Default {
            n236 = call "Stop camera acquisition.vi"("error in"=w610, "Module ID"=w608) -> ("error out"=w609:errorcluster)  [unwired: 9 in]
          }
          frame "Show video" {
            n237 = call "Start camera acquisition.vi"("error in"=w611, "Polling Time ms"=100, "Module ID"=w613) -> ("error out"=w614:errorcluster)  [unwired: 8 in]
          }
        }
      }
      frame "Error" {
        # "#CodeRecommended - If you ever change the name of this \"Error\" message, you'll need to update the name in the Check Loop Error.vi as well."
        # "#CodeRecommended - Consider creating a system for logging errors in some way. These errors are for notification purposes only. Handling of specific errors should be performed in the message frames that generated the error."
        # "Error - Display an error dialog. This message is sent by the \"Error Handler\" VIs at the end of other loops in this application."
        n238 = Variant To Data(error in=w621, type=errorcluster {"status"=FALSE, "code"=0, "source"=""} ("error constant"), Variant=w619) -> (data=w617:errorcluster, error out=w616:errorcluster)
        n239 = call <vilib>:"Simple Error Handler.vi"("error in (no error)"=w617) -> ()  [unwired: 4 in, 5 out]
        n240 = Merge Errors(w616) -> (w615:errorcluster)
      }
      frame "Confirm Quit" {
        # "#CodeNeeded - If you want to provide an \"Are you sure\" dialog (or some other notification) before the application exits, place that code here. This message is typically sent from a Panel Close? event."
        # "Confirm Quit - Message that can confirm whether or not the user wants to exit the application."
        n241 = call-poly "Enqueue Message.vi"("Priority Message? (F)"=TRUE, "error in (no error)"=w628, "Message"="Exit", "Message Queue"=w624) -> ("error out"=w625:errorcluster)  [unwired: 6 in, 1 out]
        n242 = Merge Errors(w625) -> (w626:errorcluster)
      }
      frame "Exit" {
        # "Exit - Exit the application."
        n243 = Variant To Data(type=errorcluster {"status"=FALSE, "code"=0, "source"=""} ("error constant"), Variant=w637) -> (data=w638:errorcluster)  [unwired: 1 in, 1 out]
        n244 = call <vilib>:"Simple Error Handler.vi"("error in (no error)"=w638) -> ()  [unwired: 4 in, 5 out]
        n245 = Unbundle By Name(w634) -> ("Camera Mod ID"=w630:i32, "Arduino Mod ID"=w633:i32)
        n246 = call "Fire User Event - Stop.vi"("User Event - Stop"=w642) -> ("error out"=w641:errorcluster)  [unwired: 10 in]
        n247 = Release Queue(queue=w645, error in (no error)=w640) -> (error out=w636:errorcluster)  [unwired: 1 in, 2 out]
        n248 = call "Stop motor.vi"("error in"=w636, "Module ID"=w633) -> ("error out"=w635:errorcluster)  [unwired: 9 in]
        n249 = call "Stop Module.vi"("error in"=w635, "Module ID"=w633) -> ("error out"=w632:errorcluster)  [unwired: 9 in]
        n250 = call "Disconnect.vi"("error in"=w632, "Module ID"=w630) -> ("error out"=w631:errorcluster)  [unwired: 9 in]
        n251 = call "Stop Module.vi"("error in"=w631, "Module ID"=w630) -> ("error out"=w629:errorcluster)  [unwired: 9 in]
        n252 = Merge Errors(w641, w629) -> (w643:errorcluster)
      }
      frame Default {
        # "'Default' case only runs if there is a message that isn't defined in any of the other cases.  Output a programming error."
        n253 = xnode "Error Ring"("parameter 0"=w646) -> ("error out"=w647:errorcluster)
      }
    }
    n254 = call "Error Handler - Message Handling Loop.vi"("error in (no error)"=w35, "Message Queue"=w37) -> ("dup error in"=w36:errorcluster)  [unwired: 8 in, 1 out]
  }
  n255 = while {
    tunnel: w32 -> [w662]
    shift-right: [w660] -> w28
    shift-left: w25 -> [w661]
    tunnel: [w656] -> w26
    stop <- w658 stop-if-true
    # "Event Handling Loop"
    n256 = event shown="[15] \"Start acquisition\": Value Change" {
      selector: w661 -> [_ _ _ _ _ _ _ _ _ _ _ _ _ _ _ _ _ _ _ _ _ _ _]
      dyn-events: [_ _ _ _ _ _ _ _ _ _ _ _ _ _ _ _ _ _ _ _ _ _ _] -> w660
      timeout: _ -> [_ _ _ _ _ _ _ _ _ _ _ _ _ _ _ _ _ _ _ _ _ _ _]
      tunnel: [_ _ _ _ _ _ _ _ _ _ _ _ _ TRUE ("Discard?") _ _ _ _ _ _ _ _ _] -> w658
      tunnel: w662 -> [w667 w671 w676 w681 w688 w692 w695 w701 w704 w708 w711 w712 w717 w719 w723 w727 w729 w737 w741 w748 w753 w756 w764]
      tunnel: [w666 w670 w674 w679 w686 w690 w696 w699 w702 w706 _ _ w716 _ w721 w725 w732 w735 w739 w749 w751 w757 w765] -> w659
      tunnel: [w665 w672 w675 w680 w687 w691 w694 w700 w703 w707 w711 w712 w715 w719 w722 w726 w733 w736 w740 w747 w752 w758 w763] -> w657
      event Panel Close? {
        # "Send the 'Confirm Quit' message if the user closes the panel of the VI. Discard the event so the 'Confirm Quit' message has a chance to run."
        n257 = event-data() -> ()  [unwired: 1 in, 1 out]
        n258 = call-poly "Enqueue Message.vi"("Priority Message? (F)"=TRUE, "Message"="Confirm Quit", "Message Queue"=w667) -> ("error out"=w666:errorcluster, "dup Message Queue"=w665:refnum<queue>)  [unwired: 7 in]
        n259 = event-data("Discard?"=TRUE) -> ()  [unwired: 1 in, 1 out]
      }
      event User Event {
        n260 = event-data() -> ()  [unwired: 1 in, 1 out]
        n261 = call-poly "Enqueue Message.vi"("Message"="Connect to Arduino", "Message Queue"=w671) -> ("error out"=w670:errorcluster, "dup Message Queue"=w672:refnum<queue>)  [unwired: 8 in]
      }
      event User Event {
        n262 = event-data() -> ()  [unwired: 1 in, 1 out]
        n263 = call-poly "Enqueue Message.vi"("Message"="Arduino connected", "Message Queue"=w676) -> ("error out"=w674:errorcluster, "dup Message Queue"=w675:refnum<queue>)  [unwired: 8 in]
      }
      event User Event {
        n264 = event-data() -> ()  [unwired: 1 in, 1 out]
        n265 = call-poly "Enqueue Message.vi"("Message Data"=" Arduino connection failed. Retrying..." ("Message"), "Message"="Update display", "Message Queue"=w681) -> ("error out"=w679:errorcluster, "dup Message Queue"=w680:refnum<queue>)  [unwired: 7 in]
      }
      event User Event {
        n266 = event-data() -> ("Position"=w684:i32, "End-stops"=w683:cluster{"ES1":bool, "ES2":bool})  [unwired: 1 in]
        n267 = Bundle("Position"=w684, "End-stops"=w683) -> (w682:T13)  [unwired: 1 in]
        n268 = call-poly "Enqueue Message.vi"("Message Data"=w682, "Message"="Update motor info", "Message Queue"=w688) -> ("error out"=w686:errorcluster, "dup Message Queue"=w687:refnum<queue>)  [unwired: 7 in]
      }
      event User Event {
        n269 = event-data() -> ()  [unwired: 1 in, 1 out]
        n270 = call-poly "Enqueue Message.vi"("Message"="End position reached", "Message Queue"=w692) -> ("error out"=w690:errorcluster, "dup Message Queue"=w691:refnum<queue>)  [unwired: 8 in]
      }
      event User Event {
        n271 = event-data() -> ()  [unwired: 1 in, 1 out]
        n272 = call-poly "Enqueue Message.vi"("Message"="Home reached", "Message Queue"=w695) -> ("error out"=w696:errorcluster, "dup Message Queue"=w694:refnum<queue>)  [unwired: 8 in]
      }
      event User Event {
        n273 = event-data() -> ("End-stops"=w697:cluster{"ES1":bool, "ES2":bool})  [unwired: 1 in]
        n274 = call-poly "Enqueue Message.vi"("Message Data"=w697, "Message"="End-stop reached", "Message Queue"=w701) -> ("error out"=w699:errorcluster, "dup Message Queue"=w700:refnum<queue>)  [unwired: 7 in]
      }
      event User Event {
        n275 = event-data() -> ()  [unwired: 1 in, 1 out]
        n276 = call-poly "Enqueue Message.vi"("Message"="Connect to camera", "Message Queue"=w704) -> ("error out"=w702:errorcluster, "dup Message Queue"=w703:refnum<queue>)  [unwired: 8 in]
      }
      event User Event {
        n277 = event-data() -> ()  [unwired: 1 in, 1 out]
        n278 = call-poly "Enqueue Message.vi"("Message"="Camera connected", "Message Queue"=w708) -> ("error out"=w706:errorcluster, "dup Message Queue"=w707:refnum<queue>)  [unwired: 8 in]
      }
      event User Event {
        n279 = event-data() -> ("Image"=w710:T1)  [unwired: 1 in]
        n280 = local write "Image"(w710) -> ()
      }
      event Application Instance Close {
        # "#CodeRecommended - When a project closes, all VIs within that project are aborted and leave memory. However, any code placed in this event frame is guaranteed to run to completion, so add any cleanup code that absolutely must happen here."
        n281 = event-data() -> ()  [unwired: 1 in, 1 out]
      }
      event "Exit": Value Change {
        n282 = event-data() -> ()  [unwired: 1 in, 1 out]
        n283 = call-poly "Enqueue Message.vi"("Priority Message? (F)"=TRUE, "Message"="Exit", "Message Queue"=w717) -> ("error out"=w716:errorcluster, "dup Message Queue"=w715:refnum<queue>)  [unwired: 7 in]
      }
      event User Event {
        # "The Message Handling Loop processed an \"Exit\" message, which fired this event to stop the Event Handling Loop."
        n284 = event-data() -> ()  [unwired: 1 in, 1 out]
      }
      event "Settings": Value Change {
        n285 = event-data() -> ()  [unwired: 1 in, 1 out]
        n286 = call-poly "Enqueue Message.vi"("Message"="Configuration dialog", "Message Queue"=w723) -> ("error out"=w721:errorcluster, "dup Message Queue"=w722:refnum<queue>)  [unwired: 8 in]
      }
      event "Start acquisition": Value Change {
        n287 = event-data() -> ()  [unwired: 1 in, 1 out]
        n288 = call-poly "Enqueue Message.vi"("Message"="Start acquisition", "Message Queue"=w727) -> ("error out"=w725:errorcluster, "dup Message Queue"=w726:refnum<queue>)  [unwired: 8 in]
      }
      event "Stop": Value Change {
        n289 = event-data() -> ()  [unwired: 1 in, 1 out]
        n290 = Flush Queue(queue=w729) -> (queue out=w728:refnum<queue>, error out=w730:errorcluster)  [unwired: 1 in, 1 out]
        n291 = call-poly "Enqueue Message.vi"("error in (no error)"=w730, "Message"="Stop motor", "Message Queue"=w728) -> ("error out"=w732:errorcluster, "dup Message Queue"=w733:refnum<queue>)  [unwired: 7 in]
      }
      event "Home": Value Change {
        n292 = event-data() -> ()  [unwired: 1 in, 1 out]
        n293 = call-poly "Enqueue Message.vi"("Message"="Home", "Message Queue"=w737) -> ("error out"=w735:errorcluster, "dup Message Queue"=w736:refnum<queue>)  [unwired: 8 in]
      }
      event "To Matlab": Value Change {
        n294 = event-data() -> ()  [unwired: 1 in, 1 out]
        n295 = call-poly "Enqueue Message.vi"("Message"="Export to Matlab", "Message Queue"=w741) -> ("error out"=w739:errorcluster, "dup Message Queue"=w740:refnum<queue>)  [unwired: 8 in]
      }
      event "CW Button", "CCW Button": Value Change {
        n296 = event-data() -> ()  [unwired: 1 in, 1 out]
        n297 = Select(t=Motor_direction_--_enum."CW" ("Direction"), s="CW Button", f=Motor_direction_--_enum."CCW") -> (s? t:f=w745:T4)
        n298 = call-poly "Enqueue Message.vi"("Message Data"=w745, "Message"="Jog", "Message Queue"=w748) -> ("error out"=w749:errorcluster, "dup Message Queue"=w747:refnum<queue>)  [unwired: 7 in]
      }
      event "Set zero": Value Change {
        n299 = event-data() -> ()  [unwired: 1 in, 1 out]
        n300 = call-poly "Enqueue Message.vi"("Message"="Save zero", "Message Queue"=w753) -> ("error out"=w751:errorcluster, "dup Message Queue"=w752:refnum<queue>)  [unwired: 8 in]
      }
      event "Mostrar video": Value Change {
        n301 = event-data() -> ()  [unwired: 1 in, 1 out]
        n302 = case shown="True" "Mostrar video" {
          tunnel: ["Stop video" ("Message") "Show video" ("Message")] -> w755
          frame False {
          }
          frame True {
          }
        }
        n303 = call-poly "Enqueue Message.vi"("Message Data"=w755, "Message"="Toggle video on/off", "Message Queue"=w756) -> ("error out"=w757:errorcluster, "dup Message Queue"=w758:refnum<queue>)  [unwired: 7 in]
      }
      event "Go to zero": Value Change {
        n304 = event-data() -> ()  [unwired: 1 in, 1 out]
        n305 = call "Enqueue Message (Single).vi"("Message"="Go to zero", "Message Queue"=w764) -> ("error out"=w765:errorcluster, "dup Message Queue"=w763:refnum<queue>)  [unwired: 8 in]
      }
    }
    n306 = call "Error Handler - Event Handling Loop.vi"("error in (no error)"=w659, "Message Queue"=w657) -> ("dup error in"=w656:errorcluster)  [unwired: 8 in, 1 out]
  }
  n307 = Unregister For Events(event registration refnum=w28, error in=w26) -> (error out=w29:errorcluster)
  n308 = Merge Errors(w29, w33) -> (w30:errorcluster)
  n309 = disable-structure shown="Disabled" {
    frame Disabled {
      n310 = call "Setup and move.vi"() -> ()  [unwired: 11 in, 1 out]
    }
    frame Enabled {
    }
  }
  n311 = call "Destroy User Event - Stop.vi"("error in (no error)"=w30, "User Event - Stop"=w24) -> ("error out"=w27:errorcluster)  [unwired: 9 in]
  n312 = disable-structure shown="RUN_TIME_ENGINE==True" {
    disable-tunnel: w27 -> [_ _]
    frame condition #0 (active) {
    }
    frame condition #1 {
      # "Call Quit LabVIEW if running as a built application."
      n313 = Quit LabVIEW() -> ()  [unwired: 1 in]
    }
  }
